vi "get_rotation_matrix.vi"(10 "rotation_axis":dbl[](array[numeric]), 11 "rotation_angle":dbl) -> (3 "rotation_matrix":dbl[][](array[numeric]))   [LabVIEW 2017]
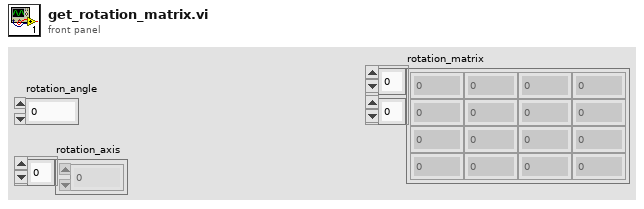
[diagram p1: front panel]
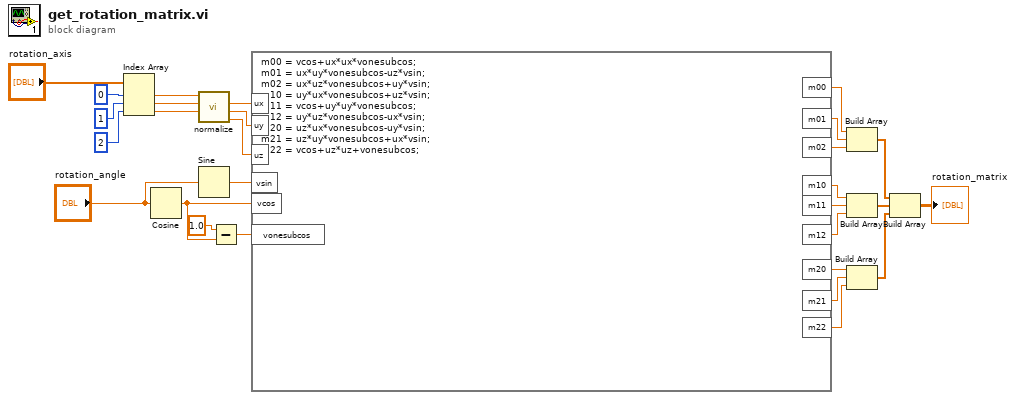
[diagram p0: block diagram]
diagram:
  n1 = Index Array(array="rotation_axis", index #1=0 ("index"), index #2=1 ("index"), index #3=2 ("index")) -> (element #1=w19:dbl, element #2=w18:dbl, element #3=w17:dbl)
  n2 = Cosine(x="rotation_angle") -> (cos(x)=w22:dbl)
  n3 = call "normalize.vi"("index2"=w17, "index1"=w18, "index0"=w19) -> ("index2"=w14:dbl, "index1"=w15:dbl, "index0"=w16:dbl)  [unwired: 5 in, 1 out]
  n4 = Sine(x="rotation_angle") -> (sin(x)=w23:dbl)
  n5 = Subtract(x=1.0, y=w22) -> (x-y=w21:dbl)
  n6 = formula code="m00 = vcos+ux*ux*vonesubcos;\nm01 = ux*uy*vonesubcos-uz*vsin;\nm02 = ux*uz*vonesubcos+uy*vsin;\nm10 = uy*ux*vonesubcos+uz*vsin;\nm11 = vcos+uy*uy*vonesubcos;\nm12 = uy*uz*vonesubcos-ux*vsin;\nm20 = uz*ux*vonesubcos-uy*vsin;\nm21 = uz*uy*vonesubcos+ux*vsin;\nm22 = vcos+uz*uz+vonesubcos;"("ux"=w16, "uy"=w15, "uz"=w14, "vsin"=w23, "vcos"=w22, "vonesubcos"=w21) -> ("m00"=w13:dbl, "m01"=w12:dbl, "m02"=w11:dbl, "m10"=w10:dbl, "m11"=w9:dbl, "m12"=w8:dbl, "m20"=w7:dbl, "m21"=w6:dbl, "m22"=w5:dbl)
  n7 = Build Array(w13, w12, w11) -> (w4:dbl[])
  n8 = Build Array(w10, w9, w8) -> (w3:dbl[])
  n9 = Build Array(w7, w6, w5) -> (w2:dbl[])
  n10 = Build Array(w4, w3, w2) -> (→"rotation_matrix":dbl[][])
